vi "solar_misc xml Parse.vi"(8 "Offset (0)":i32, 9 "Ignore Case? (T)":bool=TRUE, 10 "Tag (\"\" = Next Tag)":string, 11 "XML":string) -> (0 "Start Tag Offset":i32, 1 "Content":string, 2 "Tag":string, 3 "Remaining XML":string, 4 "Arguments (Name, Value)":string[][](array[string]))   [LabVIEW 2018]
doc: "This VI parses an xml string by tag and returns the content."
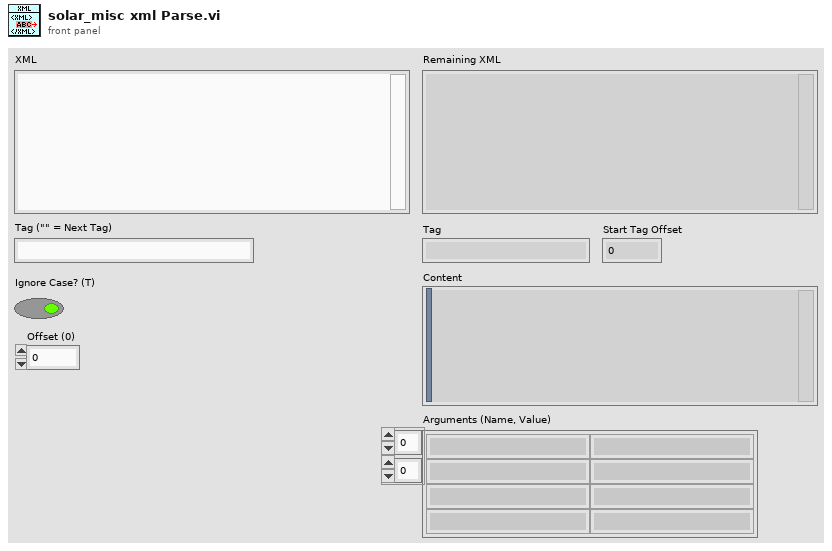
[diagram p1: front panel]
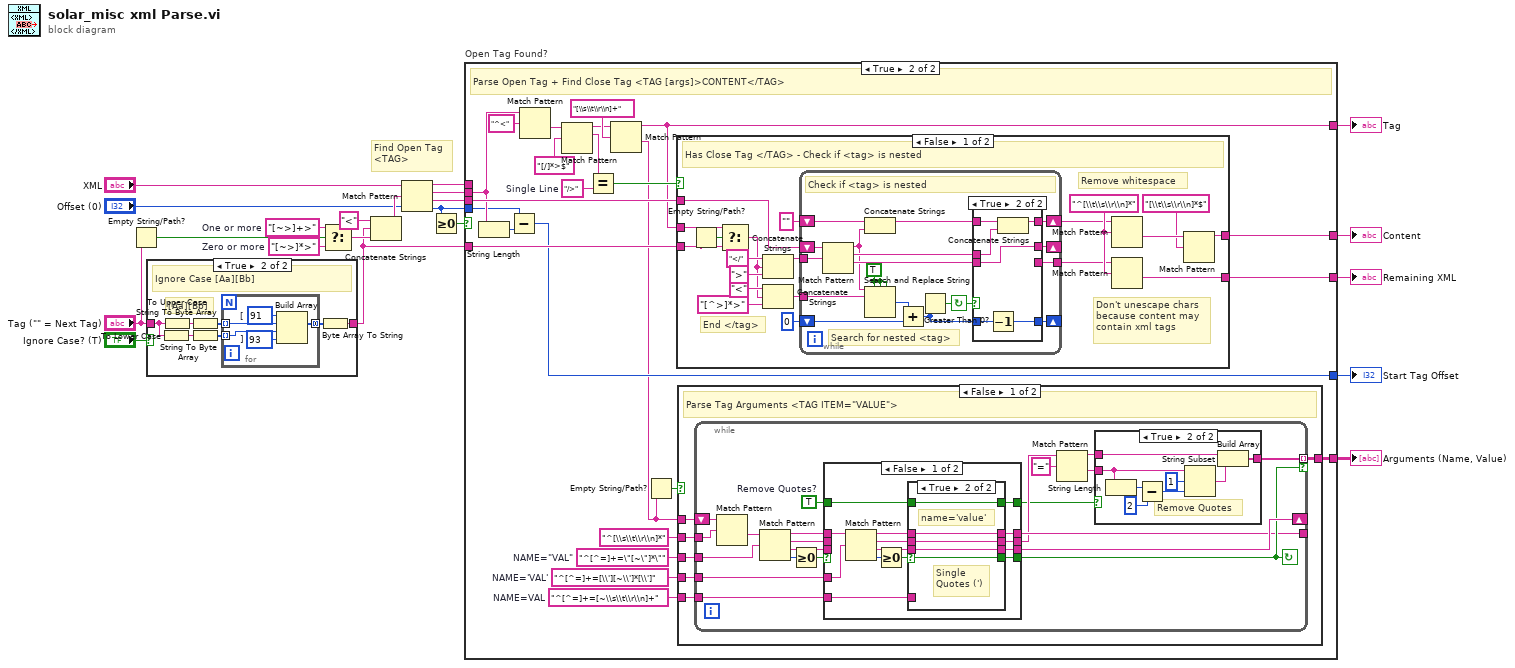
[diagram p0: block diagram]
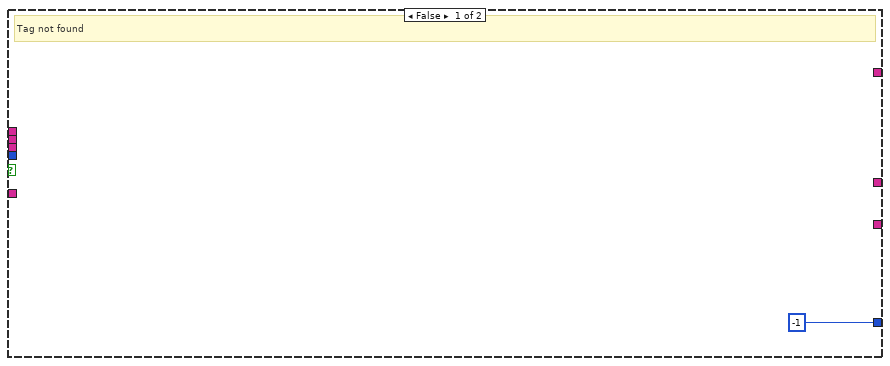
[diagram p3: hidden frame]
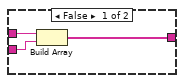
[diagram p4: hidden frame]
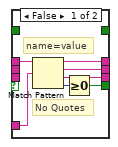
[diagram p5: hidden frame]
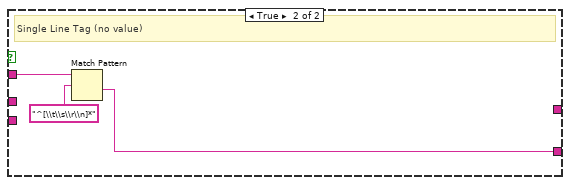
[diagram p9: hidden frame]
diagram:
  w8 = "[~>]*>"  # Zero or more
  w11 = "[~>]+>"  # One or more
  # "Find Open Tag\n<TAG>"
  n1 = Empty String/Path?(string/path="Tag (\"\" = Next Tag)") -> (empty?=w9:bool)
  n2 = case "Ignore Case?" shown="True" "Ignore Case? (T)" {
    tunnel: "Tag (\"\" = Next Tag)" -> [w22 w29]
    tunnel: [w22 w23] -> w2
    frame False {
      # "Case Sensitive"
    }
    frame True {
      # "[Aa][Bb]"
      # "Ignore Case [Aa][Bb]"
      n3 = To Lower Case(string=w29) -> (all lower case string=w27:string)
      n4 = To Upper Case(1:w29) -> (0:w28:string)
      n5 = String To Byte Array(string=w28) -> (unsigned byte array=w26:u8[])
      n6 = String To Byte Array(string=w27) -> (unsigned byte array=w25:u8[])
      n7 = for {
        tunnel: w26 -> [w34] mode=indexing
        tunnel: w25 -> [w33] mode=indexing
        tunnel: [w30] -> w24 mode=concatenating
        w31 = u8 93  # ]
        w32 = u8 91  # [
        n8 = Build Array(w32, w34, w33, w31) -> (w30:u8[])
      }
      n9 = Byte Array To String(unsigned byte array=w24) -> (string=w23:string)
    }
  }
  n10 = Select(t=w11, s=w9, f=w8) -> (s? t:f=w10:string)
  n11 = Concatenate Strings("<" ("regular expression"), w2, w10) -> (w20:string)
  n12 = Match Pattern(string="XML", regular expression=w20, offset (0)="Offset (0)") -> (before substring=w15:string, match substring=w19:string, after substring=w18:string, offset past match=w6:i32)
  n13 = Greater Or Equal To 0?(x=w6) -> (x >= 0?=w17:bool)
  n14 = case "Open Tag Found?" shown="True" w17 {
    tunnel: w19 -> [_ w46]
    tunnel: w18 -> [_ w59]
    tunnel: [_ w53] -> w16
    tunnel: w15 -> [_ _]
    tunnel: w2 -> [_ w58]
    tunnel: [_ w57] -> w14
    tunnel: [_ w40] -> w13
    tunnel: [_ w54] -> w12
    tunnel: w6 -> [_ w44]
    tunnel: [-1 w43] -> w5
    frame False {
      # "Tag not found"
    }
    frame True {
      w36 = "^[^=]+=[~\\s\\t\\r\\n]+"  # NAME=VAL
      w37 = "^[^=]+=[\\'][~\\']*[\\']"  # NAME='VAL'
      w38 = "^[^=]+=\"[~\"]*\""  # NAME="VAL"
      w48 = "/>"  # Single Line
      # "Parse Open Tag + Find Close Tag <TAG [args]>CONTENT</TAG>"
      n15 = String Length(string=w46) -> (length=w45:i32)
      n16 = Subtract(x=w44, y=w45) -> (x-y=w43:i32)
      n17 = Match Pattern(string=w46, regular expression="^<") -> (after substring=w51:string)  [unwired: 1 in, 3 out]
      n18 = Match Pattern(string=w51, regular expression="[/]*>$") -> (before substring=w50:string, match substring=w49:string)  [unwired: 1 in, 2 out]
      n19 = Equal?(x=w49, y=w48) -> (x = y?=w47:bool)
      n20 = Match Pattern(string=w50, regular expression="[\\s\\t\\r\\n]+" ("string")) -> (before substring=w40:string, after substring=w42:string)  [unwired: 1 in, 2 out]
      n21 = Empty String/Path?(string/path=w42) -> (empty?=w41:bool)
      n22 = case "Single Line Tag?" shown="False" w47 {
        tunnel: w59 -> [w132 w175]
        tunnel: [w130 w174] -> w53
        tunnel: w58 -> [w146 _]
        tunnel: [w129 _] -> w57
        tunnel: w40 -> [w147 _]
        frame False {
          w145 = "^[\\t\\s\\r\\n]*" ("regular expression")
          # "Don't unescape chars\nbecause content may\ncontain xml tags"
          # "End </tag>"
          # "Remove whitespace"
          # "Has Close Tag </TAG> - Check if <tag> is nested"
          n23 = Empty String/Path?(string/path=w146) -> (empty?=w148:bool)
          n24 = Select(t=w147, s=w148, f=w146) -> (s? t:f=w131:string)
          n25 = Concatenate Strings("</" ("regular expression"), w131, ">" ("string")) -> (w137:string)
          n26 = Concatenate Strings("<" ("string"), w131, "[^>]*>") -> (w141:string)
          n27 = while {
            tunnel: w137 -> [w165]
            tunnel: [w163] -> w134
            tunnel: w141 -> [w158]
            shift-right: [w164] -> _
            shift-left: w132 -> [w159]
            shift-right: [w160] -> w133
            shift-left: "" -> [w151]
            shift-right: [w153] -> _
            shift-left: 0 ("number of replacements") -> [w155]
            stop <- w152 continue-if-true
            w157 = TRUE ("replace all? (F)")
            # "Search for nested <tag>"
            # "Check if <tag> is nested"
            n28 = Match Pattern(string=w159, regular expression=w165) -> (before substring=w149:string, match substring=w161:string, after substring=w162:string)  [unwired: 1 in, 1 out]
            n29 = Concatenate Strings(w151, w149) -> (w150:string)
            n30 = Search and Replace String(replace all?=w157, case sensitive?=w157, multiline?=w157, input string=w149, search string=w158) -> (number of replacements=w156:i32)  [unwired: 3 in, 3 out]
            n31 = Add(x=w156, y=w155) -> (x+y=w154:i32)
            n32 = Greater Than 0?(x=w154) -> (x > 0?=w152:bool)
            n33 = case "Tag Nested?" shown="True" w152 {
              tunnel: [_ w170] -> w164
              tunnel: [w167 _] -> w163
              tunnel: w162 -> [w167 w170]
              tunnel: w161 -> [_ w173]
              tunnel: [w166 w172] -> w160
              tunnel: w150 -> [w166 w171]
              tunnel: w154 -> [_ w169]
              tunnel: [_ w168] -> w153
              frame False {
              }
              frame True {
                n34 = Decrement(x=w169) -> (x-1=w168:i32)
                n35 = Concatenate Strings(w171, w173) -> (w172:string)
              }
            }
          }
          n36 = Match Pattern(string=w133, regular expression=w145) -> (after substring=w144:string)  [unwired: 1 in, 3 out]
          n37 = Match Pattern(string=w134, regular expression=w145) -> (after substring=w130:string)  [unwired: 1 in, 3 out]
          n38 = Match Pattern(string=w144, regular expression="[\\t\\s\\r\\n]*$") -> (before substring=w129:string)  [unwired: 1 in, 3 out]
        }
        frame True {
          # "Single Line Tag (no value)"
          n39 = Match Pattern(string=w175, regular expression="^[\\t\\s\\r\\n]*") -> (after substring=w174:string)  [unwired: 1 in, 3 out]
        }
      }
      n40 = case "Has Args?" shown="False" w41 {
        tunnel: w42 -> [w65 _]
        tunnel: [w64 _] -> w54
        tunnel: "^[\\s\\t\\r\\n]*" ("regular expression") -> [w63 _]
        tunnel: w38 -> [w62 _]
        tunnel: w37 -> [w61 _]
        tunnel: w36 -> [w60 _]
        frame False {
          # "Parse Tag Arguments <TAG ITEM=\"VALUE\">"
          n41 = while {
            tunnel: [w73] -> w64 mode=indexing if=w80
            shift-right: [w81] -> _
            shift-left: w65 -> [w78]
            tunnel: [w77] -> _
            tunnel: w63 -> [w70]
            tunnel: w62 -> [w69]
            tunnel: w61 -> [w68]
            tunnel: w60 -> [w67]
            stop <- w80 continue-if-true
            w66 = TRUE  # Remove Quotes?
            # "Parse Tag Arguments <TAG ITEM=\"VALUE\">"
            n42 = Match Pattern(string=w78, regular expression=w70) -> (after substring=w79:string)  [unwired: 1 in, 3 out]
            n43 = Match Pattern(string=w79, regular expression=w69) -> (before substring=w84:string, match substring=w86:string, after substring=w82:string, offset past match=w83:i32)  [unwired: 1 in]
            n44 = Greater Or Equal To 0?(x=w83) -> (x >= 0?=w85:bool)
            n45 = case "Double Quotes?" shown="False" w85 {
              selector: w85 -> [_ w127]
              tunnel: w86 -> [_ w125]
              tunnel: [w105 w127] -> w80
              tunnel: w84 -> [w111 w126]
              tunnel: [w107 w125] -> w72
              tunnel: w82 -> [_ w128]
              tunnel: [w106 w128] -> w81
              tunnel: [w108 w126] -> w77
              tunnel: [w101 w124] -> w71
              tunnel: w66 -> [w100 w124]
              tunnel: w68 -> [w99 _]
              tunnel: w67 -> [w98 _]
              frame False {
                n46 = Match Pattern(string=w111, regular expression=w99) -> (before substring=w109:string, match substring=w103:string, after substring=w102:string, offset past match=w110:i32)  [unwired: 1 in]
                n47 = Greater Or Equal To 0?(x=w110) -> (x >= 0?=w104:bool)
                n48 = case "Single Quotes?" shown="True" w104 {
                  selector: w104 -> [_ w120]
                  tunnel: w109 -> [w117 w123]
                  tunnel: [w116 w123] -> w108
                  tunnel: [w115 w122] -> w107
                  tunnel: [w114 w121] -> w106
                  tunnel: [w113 w120] -> w105
                  tunnel: w103 -> [_ w122]
                  tunnel: w102 -> [_ w121]
                  tunnel: [_ w119] -> w101
                  tunnel: w100 -> [_ w119]
                  tunnel: w98 -> [w112 _]
                  frame False {
                    # "No Quotes"
                    # "name=value"
                    n49 = Match Pattern(string=w117, regular expression=w112) -> (before substring=w116:string, match substring=w115:string, after substring=w114:string, offset past match=w118:i32)  [unwired: 1 in]
                    n50 = Greater Or Equal To 0?(x=w118) -> (x >= 0?=w113:bool)
                  }
                  frame True {
                    # "Single\nQuotes (')"
                    # "name='value'"
                  }
                }
              }
              frame True {
                # "Double\nQuotes (\")"
                # "name=\"value\""
              }
            }
            n51 = Match Pattern(string=w72, regular expression="=") -> (before substring=w76:string, after substring=w75:string)  [unwired: 1 in, 2 out]
            n52 = case "Remove Quotes?" shown="True" w71 {
              tunnel: w76 -> [w89 w96]
              tunnel: w75 -> [w88 w92]
              tunnel: [w87 w90] -> w73
              frame False {
                n53 = Build Array(w89, w88) -> (w87:string[])
              }
              frame True {
                # "Remove Quotes"
                n54 = String Length(string=w92) -> (length=w93:i32)
                n55 = Subtract(x=w93, y=2 ("x")) -> (x-y=w94:i32)
                n56 = String Subset(string=w92, offset (0)=1, length (rest)=w94) -> (substring=w97:string)
                n57 = Build Array(w96, w97) -> (w90:string[])
              }
            }
          }
        }
        frame True {
          # "No Tag Arguments <TAG>"
        }
      }
    }
  }
  "Remaining XML" <- w16
  "Tag" <- w13
  "Arguments (Name, Value)" <- w12
  "Content" <- w14
  "Start Tag Offset" <- w5
